vi "ModAndDivide.vi"(1 "y":dbl, 2 "x":dbl) -> (0 "x%y ranged":dbl)   [LabVIEW 2019]
uses:
  448ea777-39d1-48d6-bf17-e3329b2851e8.vi
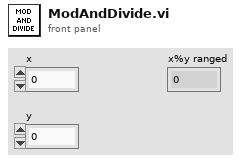
[diagram p1: front panel]
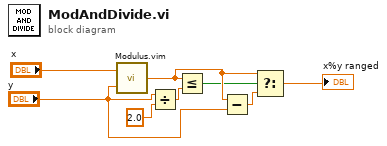
[diagram p0: block diagram]
diagram:
  n1 = call "Modulus.vim"("y"="y", "x"="x") -> ("x%y"=w8:dbl)
  n2 = Divide(x="y", y=2.0) -> (x/y=w1:dbl)
  n3 = Less Or Equal?(x=w8, y=w1) -> (x <= y?=w3:bool)
  n4 = Subtract(x=w8, y="y") -> (x-y=w4:dbl)
  n5 = Select(t=w8, s=w3, f=w4) -> (s? t:f=→"x%y ranged":dbl)
